vi "Set Socket Opt.vi"(8 "error in":errorcluster, 9 "value":variant, 10 "Socket option":T1=enum."ZMQ_SWAP", 11 "socket in":refnum<class "Socket.lvclass">) -> (0 "error out":errorcluster, 3 "socket out":refnum<class "Socket.lvclass">)   [LabVIEW 2025, in "ZeroMQ.lvlib" / "Socket.lvclass"]
doc: "Sets the specified <b>option</b> to the given <b>value</b>. The type of data connected to value must match that expected by the option (see the API documentation).\n\nNote that LabVIEW strings are used for \"raw\" data.\n\nDetailed API documentation: http://api.zeromq.org/3-2:zmq-setsockopt"
uses:
  Socket.lvclass
  libzmq-v143-mt-4_3_6/ctls/SocketOption.ctl
  Socket.lvclass/Socket.ctl
  libzmq-v143-mt-4_3_6/LibZMQ.lvlib
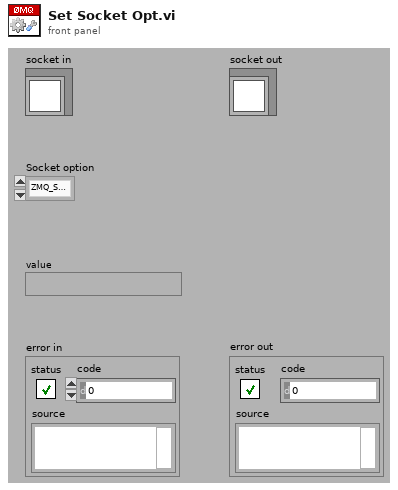
[diagram p1: front panel]
types:
  T1 = typedef "LibZMQ.lvlib/SocketOption.ctl" = enum8{"NONE", "ZMQ_HWM", "<2>", "ZMQ_SWAP", "ZMQ_AFFINITY", "ZMQ_ROUTING_ID", "ZMQ_SUBSCRIBE", "ZMQ_UNSUBSCRIBE", "ZMQ_RATE", "ZMQ_RECOVERY_IVL", "ZMQ_MCAST_LOOP", "ZMQ_SNDBUF", "ZMQ_RCVBUF", "ZMQ_RCVMORE", "ZMQ_FD", "ZMQ_EVENTS", "ZMQ_TYPE", "ZMQ_LINGER", "ZMQ_RECONNECT_IVL", "ZMQ_BACKLOG", "ZMQ_RECOVERY_IVL_MSEC", "ZMQ_RECONNECT_IVL_MAX", "ZMQ_MAXMSGSIZE", "ZMQ_SNDHWM", "ZMQ_RCVHWM", "ZMQ_MULTICAST_HOPS", "<26>", "ZMQ_RCVTIMEO", "ZMQ_SNDTIMEO", "<29>", "<30>", "ZMQ_IPV4ONLY", "ZMQ_LAST_ENDPOINT", "ZMQ_ROUTER_MANDATORY", "ZMQ_TCP_KEEPALIVE", "ZMQ_TCP_KEEPALIVE_CNT", "ZMQ_TCP_KEEPALIVE_IDLE", "ZMQ_TCP_KEEPALIVE_INTVL", "ZMQ_TCP_ACCEPT_FILTER", "ZMQ_IMMEDIATE", "ZMQ_XPUB_VERBOSE", "ZMQ_ROUTER_RAW", "ZMQ_IPV6", "ZMQ_MECHANISM", "ZMQ_PLAIN_SERVER", "ZMQ_PLAIN_USERNAME", "ZMQ_PLAIN_PASSWORD", "ZMQ_CURVE_SERVER", "ZMQ_CURVE_PUBLICKEY", "ZMQ_CURVE_SECRETKEY", "ZMQ_CURVE_SERVERKEY", "ZMQ_PROBE_ROUTER", "ZMQ_REQ_CORRELATE", "ZMQ_REQ_RELAXED", "ZMQ_CONFLATE", "ZMQ_ZAP_DOMAIN", "ZMQ_ROUTER_HANDOVER", "ZMQ_TOS", "ZMQ_IPC_FILTER_PID", "ZMQ_IPC_FILTER_UID", "ZMQ_IPC_FILTER_GID", "ZMQ_CONNECT_ROUTING_ID", "ZMQ_GSSAPI_SERVER", "ZMQ_GSSAPI_PRINCIPAL", "ZMQ_GSSAPI_SERVICE_PRINCIPAL", "ZMQ_GSSAPI_PLAINTEXT", "ZMQ_HANDSHAKE_IVL", "<67>", "ZMQ_SOCKS_PROXY", "ZMQ_XPUB_NODROP", "ZMQ_BLOCKY", "ZMQ_XPUB_MANUAL", "ZMQ_XPUB_WELCOME_MSG", "ZMQ_STREAM_NOTIFY", "ZMQ_INVERT_MATCHING", "ZMQ_HEARTBEAT_IVL", "ZMQ_HEARTBEAT_TTL", "ZMQ_HEARTBEAT_TIMEOUT", "ZMQ_XPUB_VERBOSER", "ZMQ_CONNECT_TIMEOUT", "ZMQ_TCP_MAXRT", "ZMQ_THREAD_SAFE", "<82>", "<83>", "ZMQ_MULTICAST_MAXTPDU", "ZMQ_VMCI_BUFFER_SIZE", "ZMQ_VMCI_BUFFER_MIN_SIZE", "ZMQ_VMCI_BUFFER_MAX_SIZE", "ZMQ_VMCI_CONNECT_TIMEOUT", "ZMQ_USE_FD", "ZMQ_GSSAPI_PRINCIPAL_NAMETYPE", "ZMQ_GSSAPI_SERVICE_PRINCIPAL_NAMETYPE", "ZMQ_BINDTODEVICE", "ZMQ_ZAP_ENFORCE_DOMAIN", "ZMQ_LOOPBACK_FASTPATH", "ZMQ_METADATA", "ZMQ_MULTICAST_LOOP", "ZMQ_ROUTER_NOTIFY"}
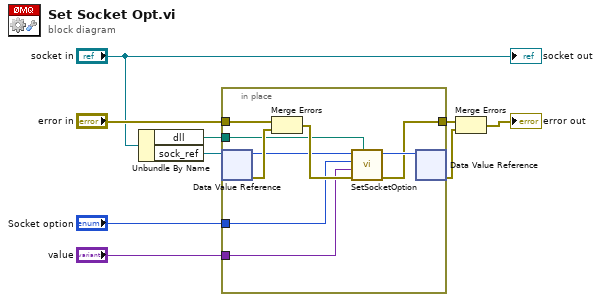
[diagram p0: block diagram]
diagram:
  n1 = Unbundle By Name("socket in") -> ("dll"=w1:path, "sock_ref"=w5:refnum<data-value>)
  n2 = in-place {
    in-place-border: [w11] -> w9
    in-place-border: "value" -> [w12]
    in-place-border: "error in" -> [w18]
    in-place-border: "Socket option" -> [w13]
    in-place-border: w1 -> [w10]
    n3 = in-place-dvr #1(w5) -> (w15:u64, w17:errorcluster)
    n4 = Merge Errors(w18, w17) -> (w16:errorcluster)
    n5 = call "SetSocketOption.vi"("path override"=w10, "error in"=w16, "value"=w12, "Socket option"=w13, "socket in"=w15) -> ("error out"=w11:errorcluster, "socket out"=w14:u64)  [unwired: 5 in]
    n6 = in-place-dvr #1(w14) -> (w3:errorcluster)  [unwired: 1 out]
  }
  n7 = Merge Errors(w9, w3) -> (→"error out":errorcluster)
  "socket out" <- "socket in"
